vi "vi.vi"() -> ()   [LabVIEW 2010]
panel:
  in  "suma":refnum<user-event>
  out "number 2":dbl
  in  "stop":bool
  in  "number":refnum<user-event>
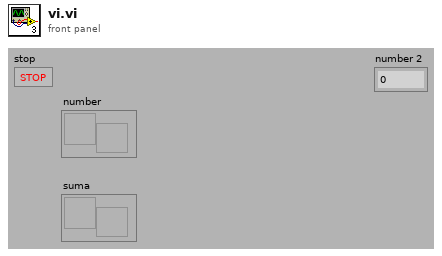
[diagram p1: front panel]
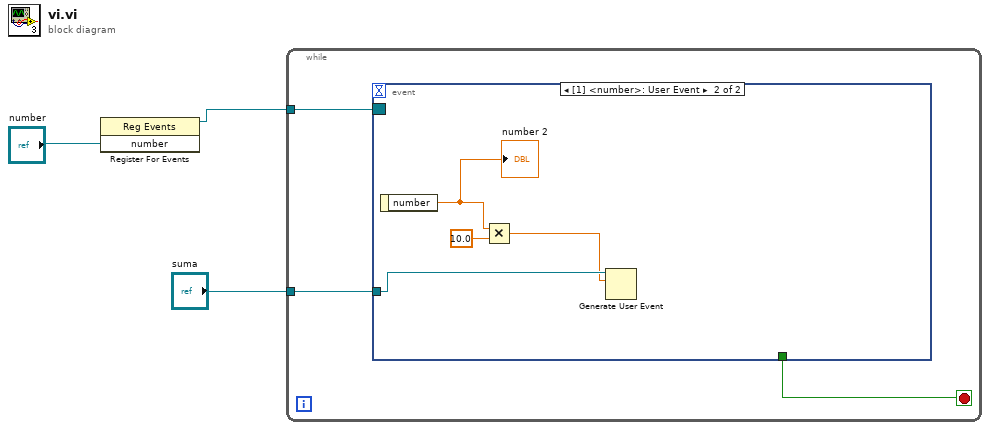
[diagram p0: block diagram]
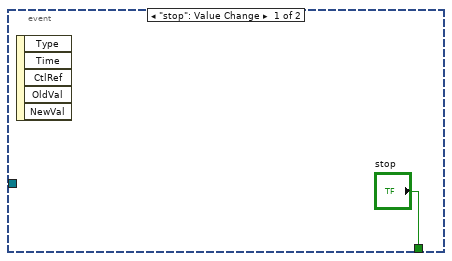
[diagram p2: hidden frame]
diagram:
  n1 = register-events("number") -> (reference out=w2:refnum<event-registration>)  [unwired: 2 in, 1 out]
  n2 = while {
    tunnel: w2 -> [w6]
    tunnel: "suma" -> [w4]
    stop <- w5 stop-if-true
    n3 = event shown="[1] <number>: User Event" {
      selector: w6 -> [_ _]
      dyn-events: _ -> [_ _]
      timeout: _ -> [_ _]
      tunnel: ["stop" _] -> w5
      tunnel: w4 -> [_ w11]
      event "stop": Value Change {
        n4 = event-data() -> ()  [unwired: 1 in, 5 out]
      }
      event User Event {
        n5 = event-data() -> ("number"=w10:dbl)  [unwired: 1 in]
        "number 2" <- w10
        n6 = Multiply(x=w10, y=10.0) -> (x*y=w8:dbl)
        n7 = Generate User Event(user event=w11, event data cluster=w8) -> ()  [unwired: 1 in, 2 out]
      }
    }
  }
